vi "Write_user_key.vi"(8 "Error in":errorcluster, 10 "Key":string, 11 "User":string) -> (0 "error out":errorcluster)   [LabVIEW 2016]
uses:
  <vilib>/Utility/config.llb/Read Key (String).vi
  <vilib>/Utility/config.llb/Write Key (String).vi
  <vilib>/Utility/config.llb/NI_LVConfig.lvlib
panel:
  in  "configuration file path":path=path "C:/Users/Lucas Oliveira/Desktop/Software_TCC/Config/Config.ini"
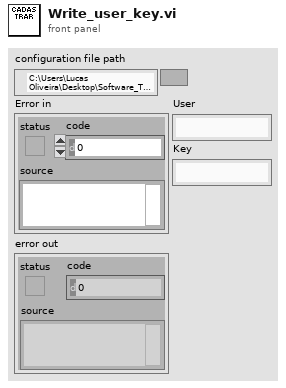
[diagram p1: front panel]
types:
  T1 = typedef "NI_LVConfig.lvlib/Config Data RefNum.ctl" = refnum<k1>
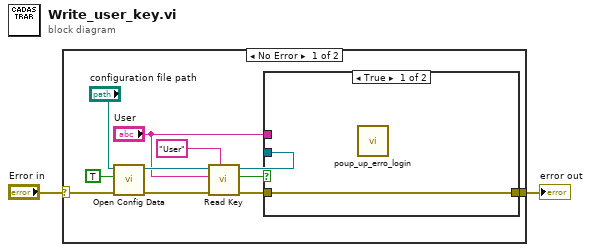
[diagram p0: block diagram]
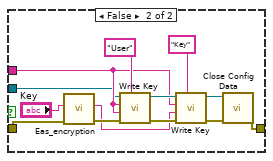
[diagram p2: hidden frame]
diagram:
  n1 = case shown="No Error" "Error in" {
    selector: "Error in" -> [w11 w28]
    tunnel: [w12 w28] -> w2
    frame No Error {
      n2 = call <vilib>:"Open Config Data.vi"("error in (no error)"=w11, "create file if necessary (T)"=TRUE, "configuration file path"="configuration file path") -> ("error out"=w9:errorcluster, "refnum"=w10:T1)  [unwired: 6 in, 1 out]
      n3 = call-poly <vilib>:"Read Key.vi"("section"="User", "error in (no error)"=w9, "key"="User", "refnum"=w10) -> ("error out"=w7:errorcluster, "found?"=w5:bool, "refnum out"=w3:T1)  [unwired: 4 in, 1 out]
      n4 = case shown="True" w5 {
        tunnel: [w14 w27] -> w12
        tunnel: w7 -> [w14 w19]
        tunnel: "User" -> [_ w17]
        tunnel: w3 -> [_ w15]
        frame True {
          n5 = call "poup_up_erro_login.vi"() -> ()  [unwired: 12 in]
        }
        frame False {
          n6 = call "Eas_encryption.vi"("error in"=w19, "Key"="Key") -> ("Error out"=w18:errorcluster, "Key"=w16:string)  [unwired: 7 in, 1 out]
          n7 = call-poly <vilib>:"Write Key.vi"("section"="User", "error in (no error)"=w18, "value"=w17, "key"=w17, "refnum"=w15) -> ("error out"=w25:errorcluster, "refnum out"=w24:T1)  [unwired: 4 in, 1 out]
          n8 = call-poly <vilib>:"Write Key.vi"("section"="Key", "error in (no error)"=w25, "value"=w16, "key"=w17, "refnum"=w24) -> ("error out"=w22:errorcluster, "refnum out"=w23:T1)  [unwired: 4 in, 1 out]
          n9 = call <vilib>:"Close Config Data.vi"("error in (no error)"=w22, "refnum"=w23) -> ("error out"=w27:errorcluster)  [unwired: 8 in, 1 out]
        }
      }
    }
    frame Error {
    }
  }
  "error out" <- w2
